vi "test_fgm_partial_pipeline.vi"() -> ()   [LabVIEW 2017, in "MPC_FXP_FGM_TestCase.lvclass"]
uses:
  MPC_FXP_FGM_TestCase.lvclass
  fpga_VIs/fixed-point/typeDefs/x_vec_type.ctl
  fpga_VIs/fixed-point/single-axis/fxp_mpc/fgm_pipiline/quadProgParams_pipe.ctl
  C:/Program Files (x86)/National Instruments/LabVIEW 2017/vi.lib/addons/_JKI Toolkits/VI Tester/TestCase.llb/TestCase.lvclass
  <vilib>/rvi/DesktopExecutionNode/Execution/niFpgaDEN_Execute.vi
  <vilib>/rvi/DesktopExecutionNode/DesktopExecutionNode.xnode
  <userlib>/_VITAC/VITAC.lvlib
panel:
  out "error out":errorcluster
  in  "Error In":errorcluster
  out "MPC_FXP_FGM_TestCase.lvclass 2":refnum<class "MPC_FXP_FGM_TestCase.lvclass">
  in  "MPC_FXP_FGM_TestCase.lvclass":refnum<class "MPC_FXP_FGM_TestCase.lvclass">
  out "all rows":dbl[][](array[numeric])
  in  "du_max":fxp<+/-,18,1>=0.197998046875
  out "QP_params":T1={"maxIter"=0, "nuN"=24, "Ns_mpc"=0, "-beta"=-0.9987945556640625, "beta+1"=1.9987945556640625}
  out "z0":dbl[](array[numeric])
  out "y0":dbl[](array[numeric])
  in  "idx2":i16
  out "x_vec":T2=[0.6000000238418579, 0.6000000238418579, -0.5999999940395355, -0.5999999940395355, 0.6000000238418579, 0.6000000238418579, 0.6000000238418579, 0.6000000238418579, -0.5999999940395355, 0.6000000238418579, -0.5999999940395355, -4.0, 0.0, 0.0, 0.0, 0.0, 0.0, 0.0, 0.0, 0.0, 0.0, 0.0, 0.0, 0.0, 0.0]
  out "yi (expected)":fxp<+/-,32,6>[](array[numeric])
  out "zi (expected)":fxp<+/-,32,6>[](array[numeric])
  out "z":fxp<+/-,32,6>[](array[numeric])
  out "y":fxp<+/-,32,6>[](array[numeric])
  in  "xk-COL":i32
  out "idx1-vec":fxp<+/-,32,2>[](array[numeric])
  out "idx2-vec":fxp<+/-,32,2>[](array[numeric])
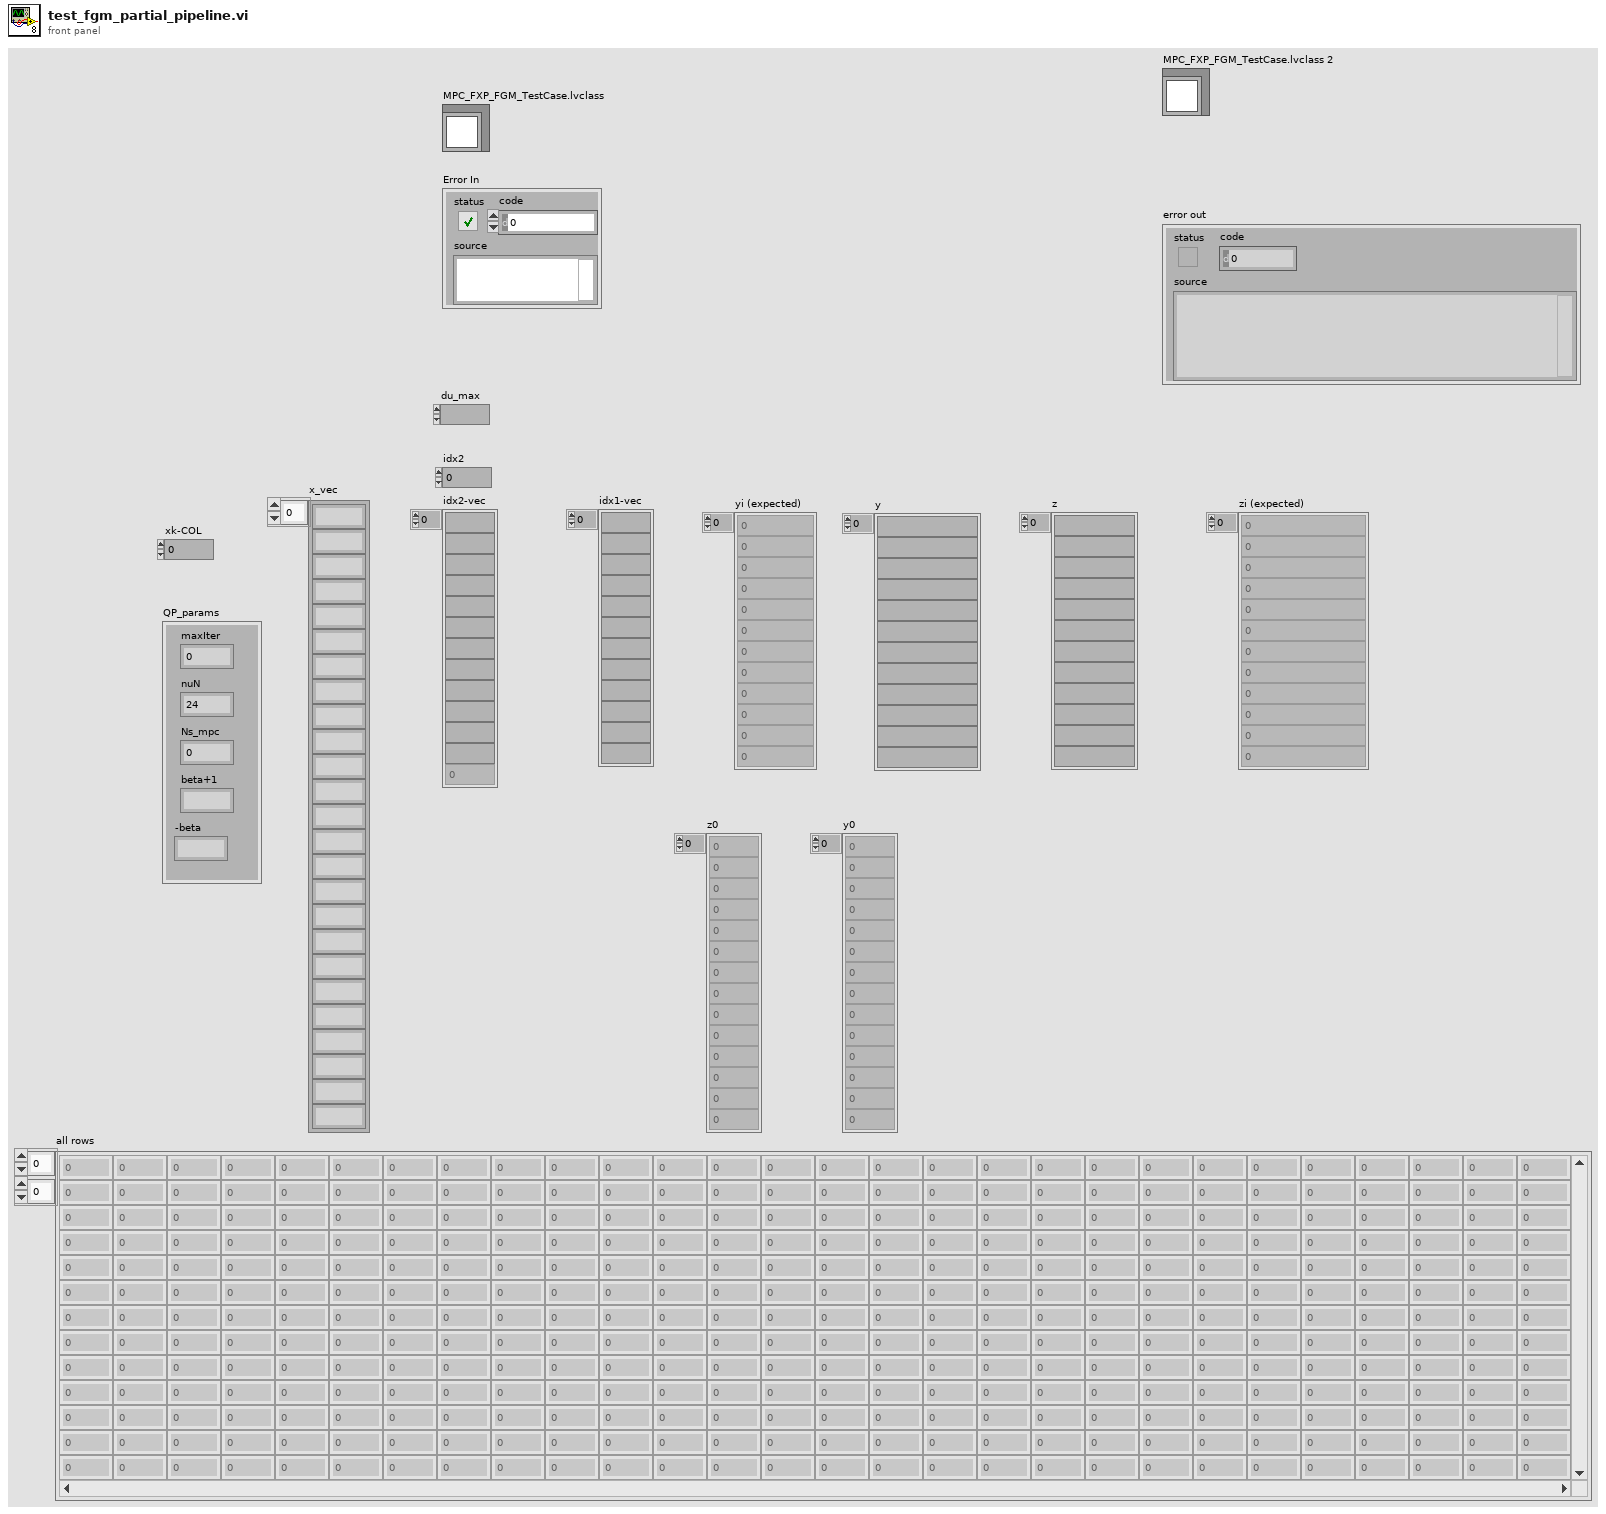
[diagram p1: front panel]
types:
  T1 = typedef "quadProgParams_pipe.ctl" = cluster{"maxIter":u16, "nuN":u16, "Ns_mpc":u16, "-beta":fxp<+/-,18,2>, "beta+1":fxp<+/-,18,2>}
  T2 = typedef "x_vec_type.ctl" = fxp<+/-,32,6>[]
  T3 = typedef "fgm_result_test_data.ctl" = cluster{"z_i_sequence":dbl[][], "y_i_sequence":dbl[][], "X_states":dbl[][]}
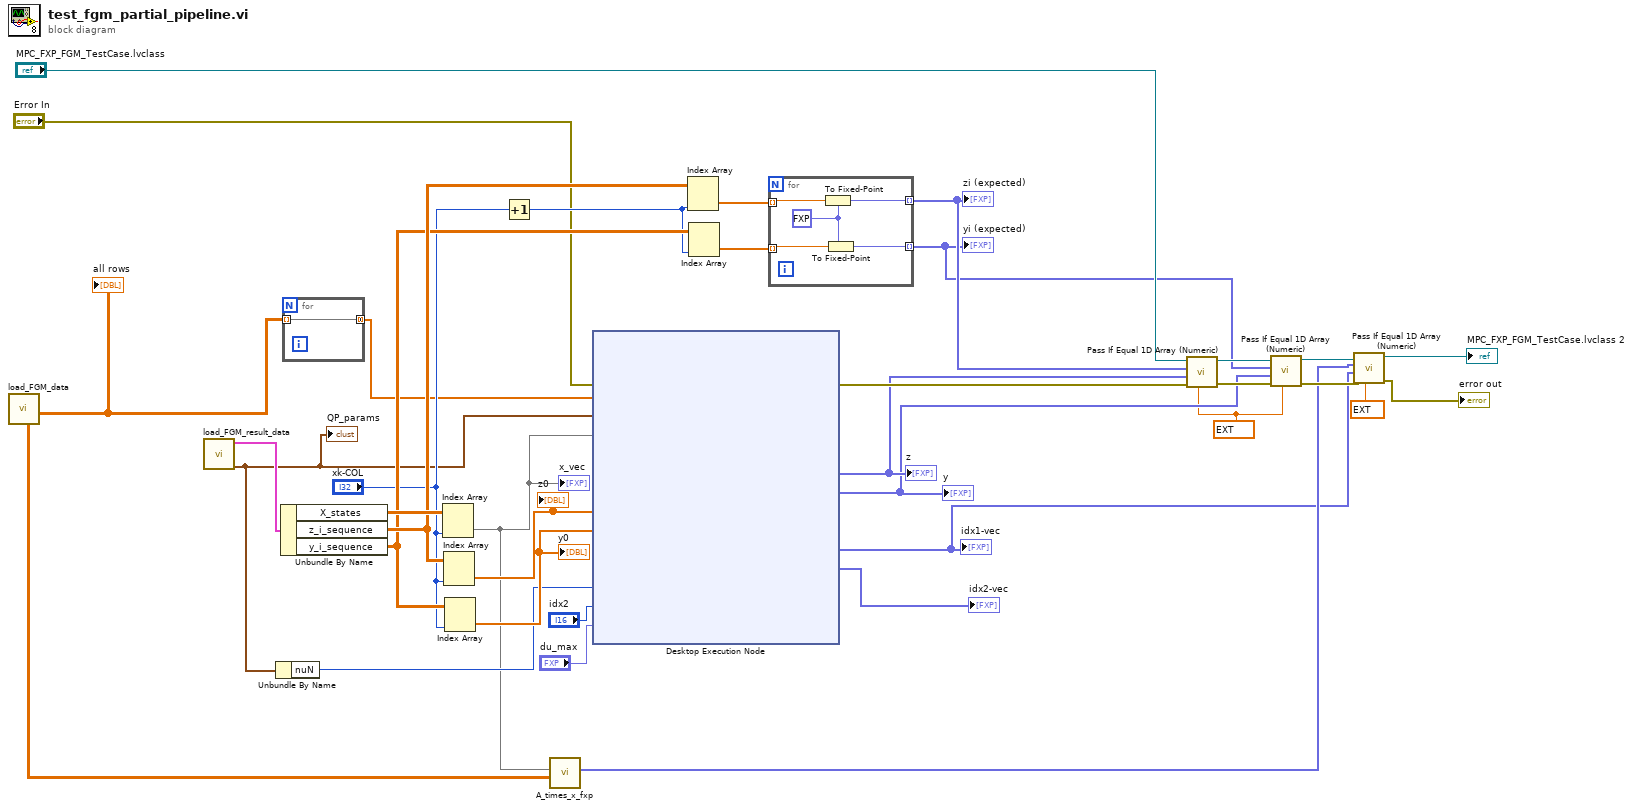
[diagram p0: block diagram]
diagram:
  w12 = ext 0.005 ("delta (optional)")
  n1 = call "load_FGM_data.vi"() -> ("all rows"=w36:dbl[][], "M"=w1:dbl[][])  [unwired: 7 in, 3 out]
  "all rows" <- w36
  n2 = call "load_FGM_result_data.vi"() -> ("QP_params"=w11:T1, "FGM_result_data"=w35:T3)  [unwired: 9 in, 1 out]
  "QP_params" <- w11
  n3 = Unbundle By Name(w11) -> ("nuN"=w10:u16)
  n4 = Unbundle By Name(w35) -> ("X_states"=w34:dbl[][], "z_i_sequence"=w33:dbl[][], "y_i_sequence"=w32:dbl[][])
  n5 = for {
    tunnel: [w37] -> w29 mode=concatenating
    tunnel: w36 -> [w37] mode=indexing
  }
  n6 = Index Array(array=w34, index (col)="xk-COL") -> (element=w2:dbl[])  [unwired: 1 in]
  "x_vec" <- w2
  n7 = Index Array(array=w33, index (col)="xk-COL") -> (element=w28:dbl[])  [unwired: 1 in]
  "z0" <- w28
  n8 = Index Array(array=w32, index (col)="xk-COL") -> (element=w27:dbl[])  [unwired: 1 in]
  "y0" <- w27
  n9 = Increment(x="xk-COL") -> (x+1=w30:i32)
  n10 = call "A_times_x_fxp.vi"("Az_mat in"=w1, "x_k"=w2) -> ("A*x"=w6:fxp<+/-,64,12>[])  [unwired: 8 in, 1 out]
  n11 = xnode "Desktop Execution Node"("Error In"="Error In", "big_mat_data"=w29, "QP_params"=w11, "x"=w2, "z0"=w28, "y0"=w27, "idx1"=w10, "idx2"="idx2", "du_max"="du_max") -> ("Error Out"=w20:errorcluster, "z"=w17:fxp<+/-,32,6>[], "y"=w13:fxp<+/-,32,6>[], "idx1"=w5:fxp<+/-,32,6>[], "idx2"=→"idx2-vec":fxp<+/-,32,6>[])  [unwired: 1 out]
  "idx1-vec" <- w5
  "y" <- w13
  "z" <- w17
  n12 = Index Array(array=w33, index (col)=w30) -> (element=w23:dbl[])  [unwired: 1 in]
  n13 = Index Array(array=w32, index (col)=w30) -> (element=w22:dbl[])  [unwired: 1 in]
  n14 = for {
    tunnel: w23 -> [w42] mode=indexing
    tunnel: w22 -> [w40] mode=indexing
    tunnel: [w41] -> w18 mode=indexing
    tunnel: [w39] -> w14 mode=indexing
    w38 = fxp<+/-,32,6> 0.0 ("fixed-point type")
    n15 = To Fixed-Point(fixed-point type=w38, number=w42) -> (fixed-point=w41:fxp<+/-,32,6>)
    n16 = To Fixed-Point(fixed-point type=w38, number=w40) -> (fixed-point=w39:fxp<+/-,32,6>)
  }
  "zi (expected)" <- w18
  "yi (expected)" <- w14
  n17 = call <userlib>:"Pass If Equal 1D Array (Numeric).vi"("delta (optional)"=w12, "error in (no error)"=w20, "actual"=w17, "expected"=w18, "TestCase in"="MPC_FXP_FGM_TestCase.lvclass") -> ("error out"=w15:errorcluster, "TestCase out"=w16:refnum<class "MPC_FXP_FGM_TestCase.lvclass">)  [unwired: 5 in]
  n18 = call <userlib>:"Pass If Equal 1D Array (Numeric).vi"("delta (optional)"=w12, "error in (no error)"=w15, "actual"=w13, "expected"=w14, "TestCase in"=w16) -> ("error out"=w7:errorcluster, "TestCase out"=w9:refnum<class "MPC_FXP_FGM_TestCase.lvclass">)  [unwired: 5 in]
  n19 = call <userlib>:"Pass If Equal 1D Array (Numeric).vi"("delta (optional)"=ext 0.00001, "error in (no error)"=w7, "actual"=w5, "expected"=w6, "TestCase in"=w9) -> ("error out"=→"error out":errorcluster, "TestCase out"=→"MPC_FXP_FGM_TestCase.lvclass 2":refnum<class "MPC_FXP_FGM_TestCase.lvclass">)  [unwired: 5 in]
